vi "moveTo_rel_XY.vi"(7 "blocking?":bool, 8 "error in":errorcluster, 10 "XYZ location (steps)":i32[](array[numeric]), 11 "Actuator cluster in":T1={"Actuator COM"="COM14", "Actuator type"=enum."Scientifica"}) -> (0 "error out":errorcluster, 3 "Actuator cluster out":T1={"Actuator COM"="COM14", "Actuator type"=enum."Scientifica"})   [LabVIEW 2015]
uses:
  controls/scientifica_commands.ctl
  controls/actuator_type.ctl
  controls/actuator_cluster.ctl
panel:
  out "response":string
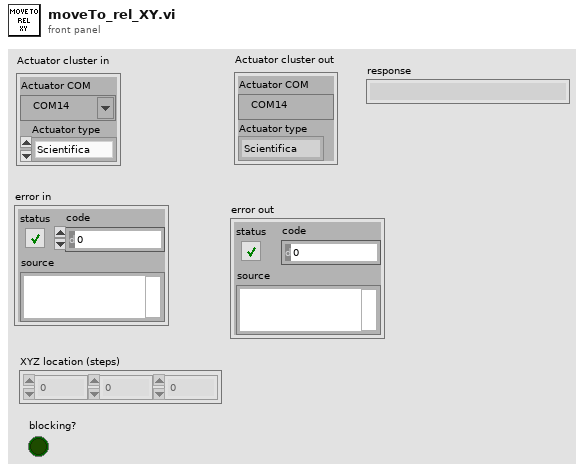
[diagram p1: front panel]
types:
  T1 = typedef "actuator_cluster.ctl" = cluster{"Actuator COM":refnum<visa-resource-name>, "Actuator type":T2}
  T2 = typedef "actuator_type.ctl" = enum16{"Scientifica", "Sutter", "Demo", "Off"}
  T3 = typedef "scientifica_commands.ctl" = enum16{"ANGLE", "INSET", "FIRST", "ZERO", "Pz", "P", "absz", "ACC", "TOP", "STOP", "rel", "relz", "abs", "IN", "vj", "APROACH", "OBJS", "OBJU", "OUT", "OBJ", "OBJL", "SET", "OBJD", "STEP", "SETSTEP", "S", "UUX", "UUY", "UUZ"}
  T4 = enum16{"READY", "ABSOLUTE MOVE", "RELATIVE MOVE", "HOMING", "WAITING", "CANCELING"}
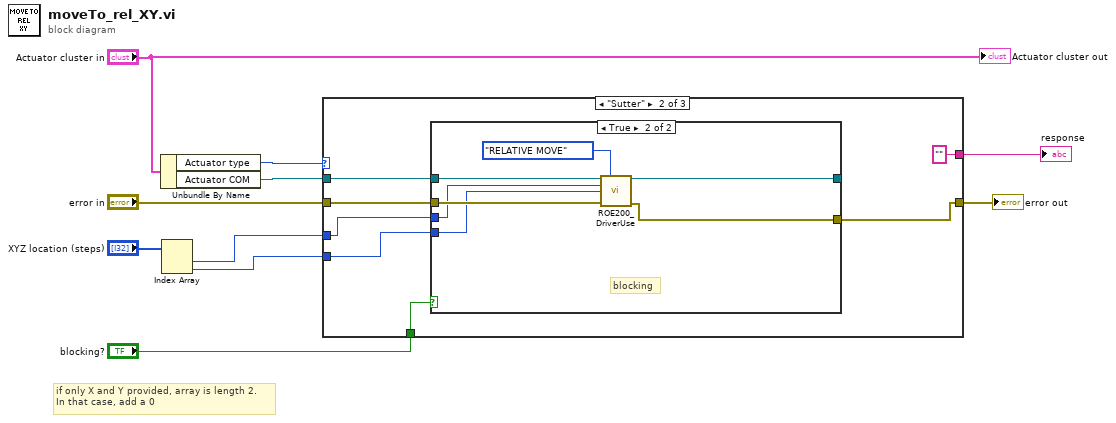
[diagram p0: block diagram]
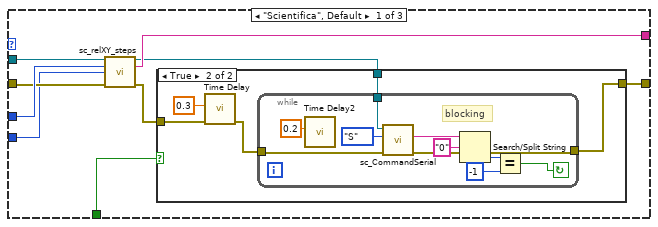
[diagram p2: hidden frame]
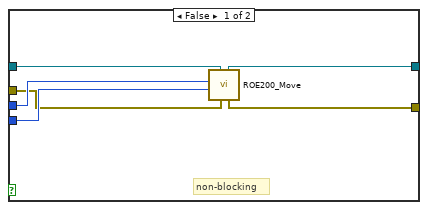
[diagram p4: hidden frame]
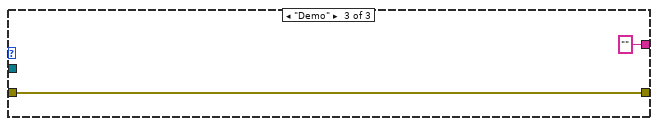
[diagram p5: hidden frame]
diagram:
  # "if only X and Y provided, array is length 2.\nIn that case, add a 0"
  n1 = Unbundle By Name("Actuator cluster in") -> ("Actuator type"=w10:T2, "Actuator COM"=w8:refnum<visa-resource-name>)
  n2 = Index Array(array="XYZ location (steps)") -> (element #1=w4:i32, element #2=w3:i32)  [unwired: 2 in]
  n3 = case shown="\"Sutter\"" w10 {
    tunnel: "error in" -> [w17 w41 w56]
    tunnel: w8 -> [w19 w42 _]
    tunnel: [w13 w37 w56] -> w6
    tunnel: w4 -> [w18 w40 _]
    tunnel: w3 -> [w11 w38 _]
    tunnel: [w16 "" ("argument integer string") "" ("argument integer string")] -> w5
    tunnel: "blocking?" -> [w15 w39 _]
    frame "Scientifica", Default {
      n4 = call "sc_relXY_steps.vi"("VISA handle"=w19, "rel X dist (steps)"=w18, "rel Y dist (steps)"=w11, "error in (no error)"=w17) -> ("Dup. VISA handle"=w12:refnum<visa-resource-name>, "Response"=w16:string, "error out"=w14:errorcluster)  [unwired: 9 in]
      n5 = case shown="True" w15 {
        tunnel: w14 -> [w20 w24]
        tunnel: [w20 w22] -> w13
        tunnel: w12 -> [_ w21]
        frame False {
        }
        frame True {
          n6 = call "Time Delay"("error in (no error)"=w24, "Delay Time (s)"=0.3) -> ("error out"=w23:errorcluster)  [unwired: 9 in]
          n7 = while {
            tunnel: w23 -> [w34]
            tunnel: [w28] -> w22
            tunnel: w21 -> [w26]
            stop <- w29 continue-if-true
            # "blocking"
            n8 = call "Time Delay2"("Delay Time (s)"=0.2) -> ()  [unwired: 10 in, 1 out]
            n9 = call "sc_CommandSerial.vi"("error in (no error)"=w34, "Scientifica commands"=scientifica_commands."S", "VISA handle"=w26) -> ("error out"=w28:errorcluster, "Response"=w32:string)  [unwired: 5 in, 2 out]
            n10 = Search/Split String(string=w32, search string/char (-)="0") -> (offset of match=w31:i32)  [unwired: 1 in, 2 out]
            n11 = Equal?(x=w31, y=-1) -> (x = y?=w29:bool)
          }
        }
      }
    }
    frame "Sutter" {
      n12 = case shown="True" w39 {
        tunnel: w42 -> [w48 w55]
        tunnel: w41 -> [w44 w54]
        tunnel: w40 -> [w47 w53]
        tunnel: w38 -> [w46 w52]
        tunnel: [w45 w50] -> _
        tunnel: [w43 w49] -> w37
        frame False {
          # "non-blocking"
          n13 = call "ROE200_Move.vi"("error in (no error)"=w44, "VISA resource name 2"=w48, "Y"=w46, "X"=w47) -> ("error out"=w43:errorcluster, "VISA resource name out"=w45:refnum<visa-resource-name>)  [unwired: 6 in]
        }
        frame True {
          # "blocking"
          n14 = call "ROE200_DriverUse.vi"("VISA resource name In"=w55, "CMD"=T4."RELATIVE MOVE", "X"=w53, "Y"=w52, "error in"=w54) -> ("VISA resource name out"=w50:refnum<visa-resource-name>, "error out"=w49:errorcluster)  [unwired: 6 in, 3 out]
        }
      }
    }
    frame "Demo" {
    }
  }
  "error out" <- w6
  "response" <- w5
  "Actuator cluster out" <- "Actuator cluster in"
